vi "Configure PA MESSAGE.vi"(8 "error in (no error)":errorcluster, 9 "Message":string, 11 "VISA resource in":refnum<visa-resource-name>) -> (0 "error out":errorcluster, 3 "VISA resource out":refnum<visa-resource-name>)   [LabVIEW 2025]
uses:
  <instrlib>/Chroma 19052/Chroma 19052.lvlib
  <instrlib>/Chroma 19052/Public/Utility/Type Def/steps--numeric.ctl
panel:
  in  "Step":T1=1 min=1 max=99 step=1
  # "Set PA Message"
  # "min 1 char, Max 15 char"
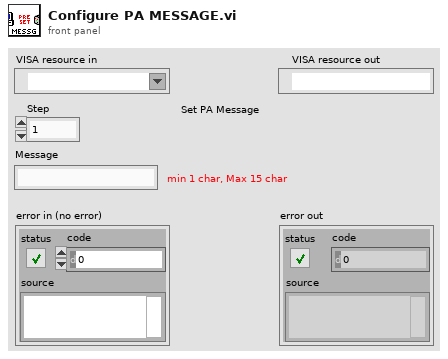
[diagram p1: front panel]
types:
  T1 = typedef "Chroma 19052.lvlib/steps--numeric.ctl" = u8
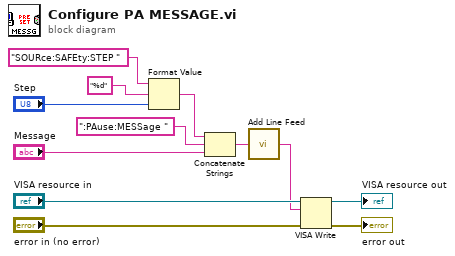
[diagram p0: block diagram]
diagram:
  n1 = Format Value(string ("")="SOURce:SAFEty:STEP ", format string="%d", value (0)="Step") -> (output string=w5:string)
  n2 = Concatenate Strings(w5, ":PAuse:MESSage ", "Message") -> (w3:string)
  n3 = call <instrlib>:"Add Line Feed.vi"("Command string"=w3) -> ("Concatenated string"=w2:string)  [unwired: 4 in]
  n4 = VISA Write(VISA resource name="VISA resource in", write buffer=w2, error in (no error)="error in (no error)") -> (VISA resource name out=→"VISA resource out":refnum<visa-resource-name>, error out=→"error out":errorcluster)  [unwired: 1 out]
